vi "sub_vi_arduino_com_port_popup.vi"() -> (18 "Arduino COM port 2":refnum<visa-resource-name>="COM6")   [LabVIEW 2016]
doc: "Displays a standard dialog box that prompts users to enter information, such as a user name and password.\n--------------------\n\nThis Express VI is configured as follows:\n\nMessage to Display to the User:\nThe inputs are:"
panel:
  in  "OK Button":bool
  in  "Arduino COM port":refnum<visa-resource-name>="COM6"
  # "Choose Arduino COM port"
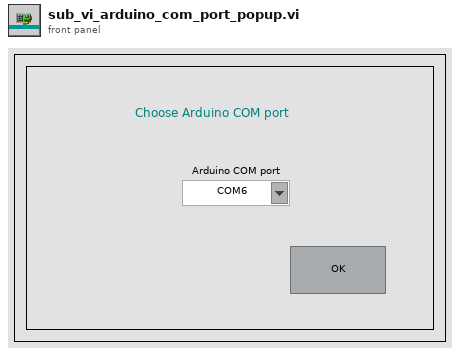
[diagram p1: front panel]
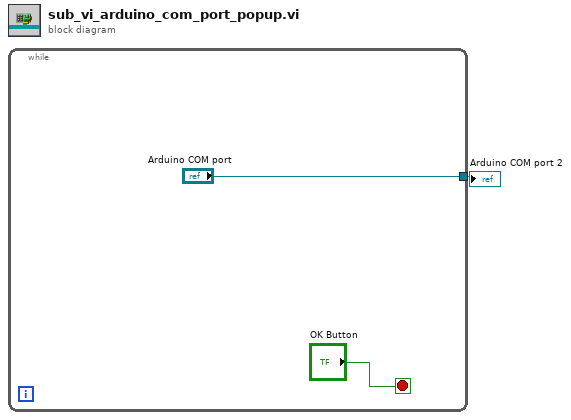
[diagram p0: block diagram]
diagram:
  n1 = while {
    tunnel: ["Arduino COM port"] -> w1
    stop <- "OK Button" stop-if-true
  }
  "Arduino COM port 2" <- w1
